vi "poly_trim(s)_xwav(s).vi"(8 "Error in":errorcluster caption="Error in (no error)", 9 "end x (end)":dbl=inf, 10 "start x (start)":dbl=-inf, 11 "xwave in":T1={"attributes"=variant, "X"={"start"=0.0, "delta"=0.0, "units"="index", "dim"="au"}, "Y"={"data"=[], "units"="au"}}) -> (0 "Error out":errorcluster, 1 "actual end x index":i32, 2 "actual start x index":i32, 3 "xwave out":T1={"attributes"=variant, "X"={"start"=0.0, "delta"=0.0, "units"="index", "dim"="au"}, "Y"={"data"=[], "units"="au"}})   [LabVIEW 2015, in "_xwav_polys.lvlib"]
uses:
  _xwav_polys.lvlib
  xwav.ctl
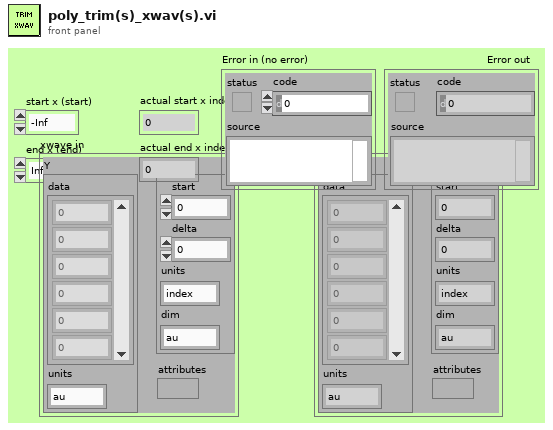
[diagram p1: front panel]
types:
  T1 = typedef "xwav.ctl" = cluster{"attributes":variant, "X":cluster{"start":dbl, "delta":dbl, "units":string, "dim":string}, "Y":cluster{"data":dbl[], "units":string}}
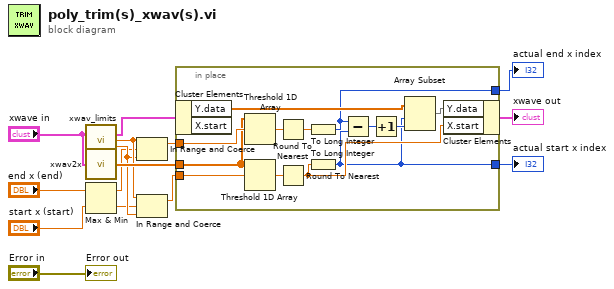
[diagram p0: block diagram]
diagram:
  n1 = call "xwav_limits.vi"("xwave"="xwave in") -> ("dup xwave"=w10:T1, "x start"=w6:dbl, "x end"=w5:dbl)  [unwired: 12 in]
  n2 = call "xwav2x.vi"("xwave"="xwave in") -> ("X"=w12:dbl[])  [unwired: 4 in]
  n3 = Max & Min(x="end x (end)", y="start x (start)") -> (max(x,y)=w4:dbl, min(x,y)=w3:dbl)
  n4 = In Range and Coerce(upper limit=w6, x=w4, lower limit=w5) -> (coerced(x)=w11:dbl)  [unwired: 1 out]
  n5 = In Range and Coerce(upper limit=w6, x=w3, lower limit=w5) -> (coerced(x)=w2:dbl)  [unwired: 1 out]
  n6 = in-place {
    in-place-border: w2 -> [w28]
    in-place-border: w11 -> [w27]
    in-place-border: w12 -> [w25]
    in-place-border: [w16] -> w9
    in-place-border: [w17] -> w8
    n7 = in-place-cluster #1(w10) -> ("Y.data"=w20:dbl[])  [unwired: 1 out]
    n8 = Threshold 1D Array(2:w27, 3:w25) -> (0:w23:dbl)  [unwired: 1 in]
    n9 = Threshold 1D Array(2:w28, 3:w25) -> (0:w24:dbl)  [unwired: 1 in]
    n10 = Round To Nearest(number=w23) -> (nearest integer value=w21:dbl)
    n11 = Round To Nearest(number=w24) -> (nearest integer value=w22:dbl)
    n12 = To Long Integer(number=w21) -> (32bit integer=w17:i32)
    n13 = To Long Integer(number=w22) -> (32bit integer=w16:i32)
    n14 = Subtract(x=w17, y=w16) -> (x-y=w19:i32)
    n15 = Increment(x=w19) -> (x+1=w18:i32)
    n16 = Array Subset(array=w20, index=w16, length=w18) -> (w26:dbl[])
    n17 = in-place-cluster #1("Y.data"=w26, "X.start"=w22) -> (→"xwave out":T1)
  }
  "actual start x index" <- w9
  "actual end x index" <- w8
  "Error out" <- "Error in"
